vi "Servo and moisture.vi"() -> (0 "LOW MOISTURE":bool, 1 "INTERMEDIATE MOISTURE":bool, 2 "HIGH MOISTURE":bool, 3 "MOISTURE LEVEL(ppm)":dbl)   [LabVIEW 2013]
uses:
  <vilib>/myRIO/Common/Instrument Driver Framework/myRIO v1.0/PWM/vis/myRIO v1.1 Open PWM.vi
  <vilib>/myRIO/Common/Instrument Driver Framework/Utilities/vis/Validate Channels.vi
  <vilib>/myRIO/Common/Instrument Driver Framework/myRIO v1.0/PWM/vis/myRIO v1.0 Reserve PWM.vi
  <vilib>/myRIO/Common/Instrument Driver Framework/myRIO v1.0/PWM/vis/myRIO v1.0 Build MUX Configuration PWM.vi
  <vilib>/myRIO/Common/Instrument Driver Framework/myRIO v1.0/Resource Manager/vis/myRIO v1.0 Reserve Channel List.vi
  <vilib>/myRIO/Common/Instrument Driver Framework/myRIO v1.0/Resource Manager/vis/myRIO v1.0 Create Configuration List.vi
  <vilib>/myRIO/Common/Instrument Driver Framework/myRIO v1.0/Resource Manager/vis/myRIO v1.0 Reserve Channel.vi
  <vilib>/myRIO/Common/Instrument Driver Framework/myRIO v1.0/Resource Manager/vis/myRIO v1.0 Unreserve Channel.vi
  <vilib>/myRIO/Common/Instrument Driver Framework/myRIO v1.0/Resource Manager/vis/myRIO v1.0 Build Mutex Name.vi
  <vilib>/myRIO/Common/Instrument Driver Framework/myRIO v1.0/myRIO v1.1 Open.vi
  <vilib>/Utility/VariantDataType/GetNumericInfo.vi
  <vilib>/Utility/error.llb/Error Cluster From Error Code.vi
  <vilib>/myRIO/Common/Instrument Driver Framework/Utilities/vis/IO Manager.vi
  <vilib>/myRIO/Common/Instrument Driver Framework/Utilities/vis/Configuration Manager.vi
  <vilib>/myRIO/Common/Instrument Driver Framework/myRIO v1.0/Resource Manager/vis/myRIO v1.0 Configure IO.vi
  <vilib>/myRIO/Common/Instrument Driver Framework/myRIO v1.0/myRIO v1.0 Close.vi
  <vilib>/myRIO/Common/Instrument Driver Framework/myRIO v1.0/PWM/vis/myRIO v1.0 Write PWM.vi
  <vilib>/myRIO/Instrument Drivers/Onboard IO/PWM/PWM.lvlib
panel:
  in  "null offset":bool
  in  "freq [Hz] 2":dbl=50.0
  out "pulse width [ms] 2":dbl=1.5
  out "duty cycle [%] 2":dbl
  in  "null offset 2":bool
  out "offset [%FS] 2":dbl
  in  "PWM channel":tag="B/PWM0"
  in  "freq [Hz]":dbl=50.0
  out "pulse width [ms]":dbl=1.5
  out "duty cycle [%]":dbl
  out "offset [%FS]":dbl
  out "x+y":dbl
  # "SERVO"
  # "MOISTURE"
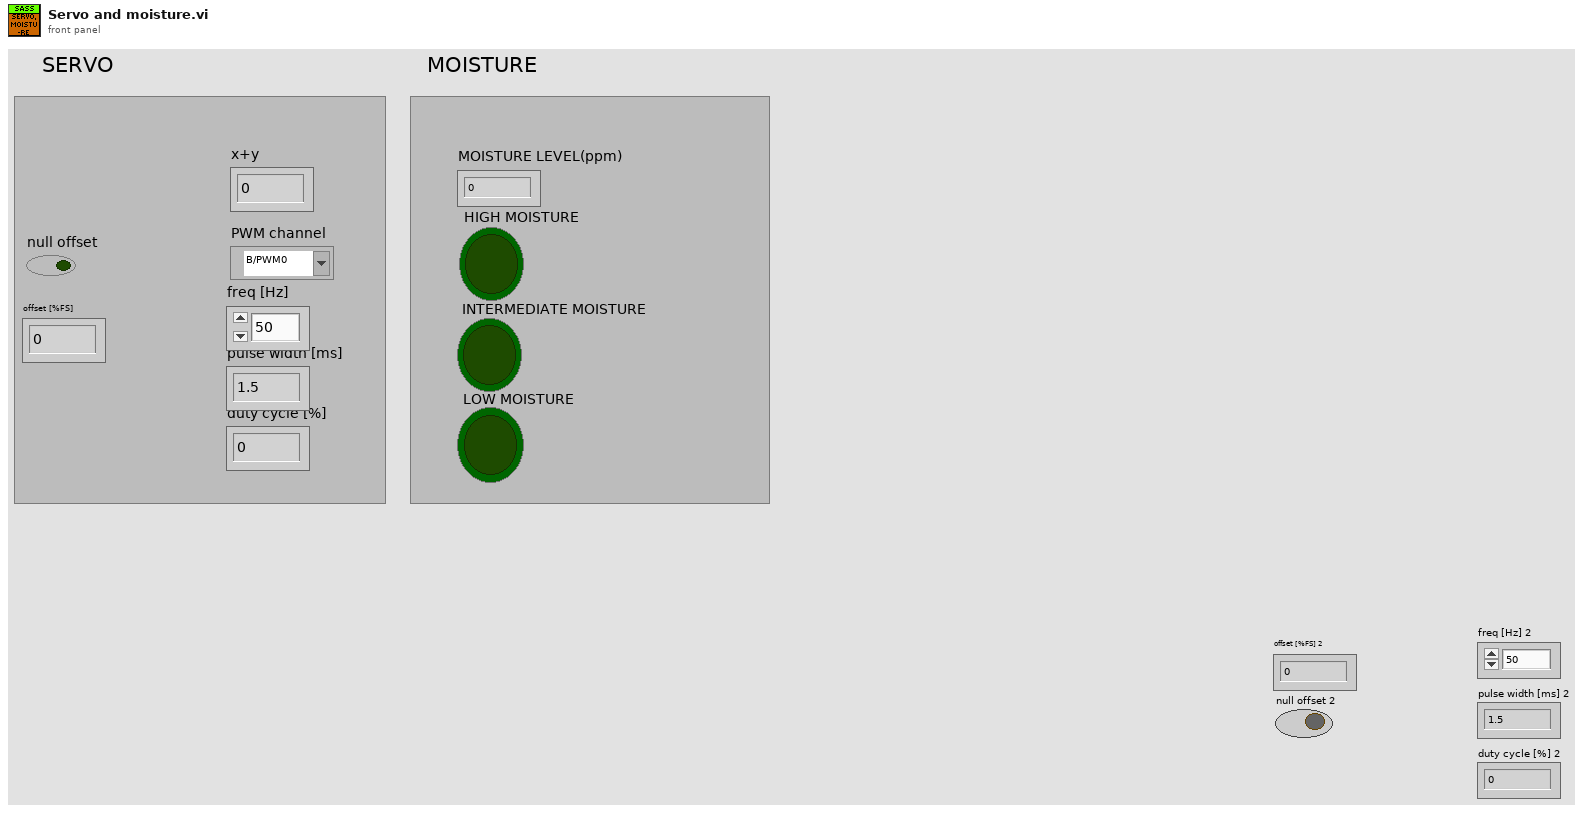
[diagram p1: front panel]
types:
  T1 = typedef "PWM.lvlib/PWM Reference.ctl" = cluster{"myRIO Reference":T2, "PWM Channels Enum":T6, "PWM Configuration":T7}
  T2 = typedef "myRIO Generic Hardware Reference.ctl" = cluster{"myRIO Model":T3, "myRIO Hardware Reference":T4}
  T3 = typedef "Hardware Version Enum.ctl" = enum16{"Unknown", "myRIO-1900", "myRIO-1950"}
  T4 = typedef "myRIO v1.0 Reference.ctl" = cluster{"Generic FPGA Reference":T5, "Allow multiple opens":bool}
  T5 = typedef "Generic FPGA Reference.ctl" = refnum<k20>
  T6 = typedef "PWM Channels Enum.ctl" = enum16{"Not Connected", "C/PWM0", "C/PWM1", "A/PWM0", "A/PWM1", "A/PWM2", "B/PWM0", "B/PWM1", "B/PWM2"}
  T7 = typedef "PWM.lvlib/PWM Configuration.ctl" = cluster{"Frequency":dbl, "Duty Cycle":dbl}
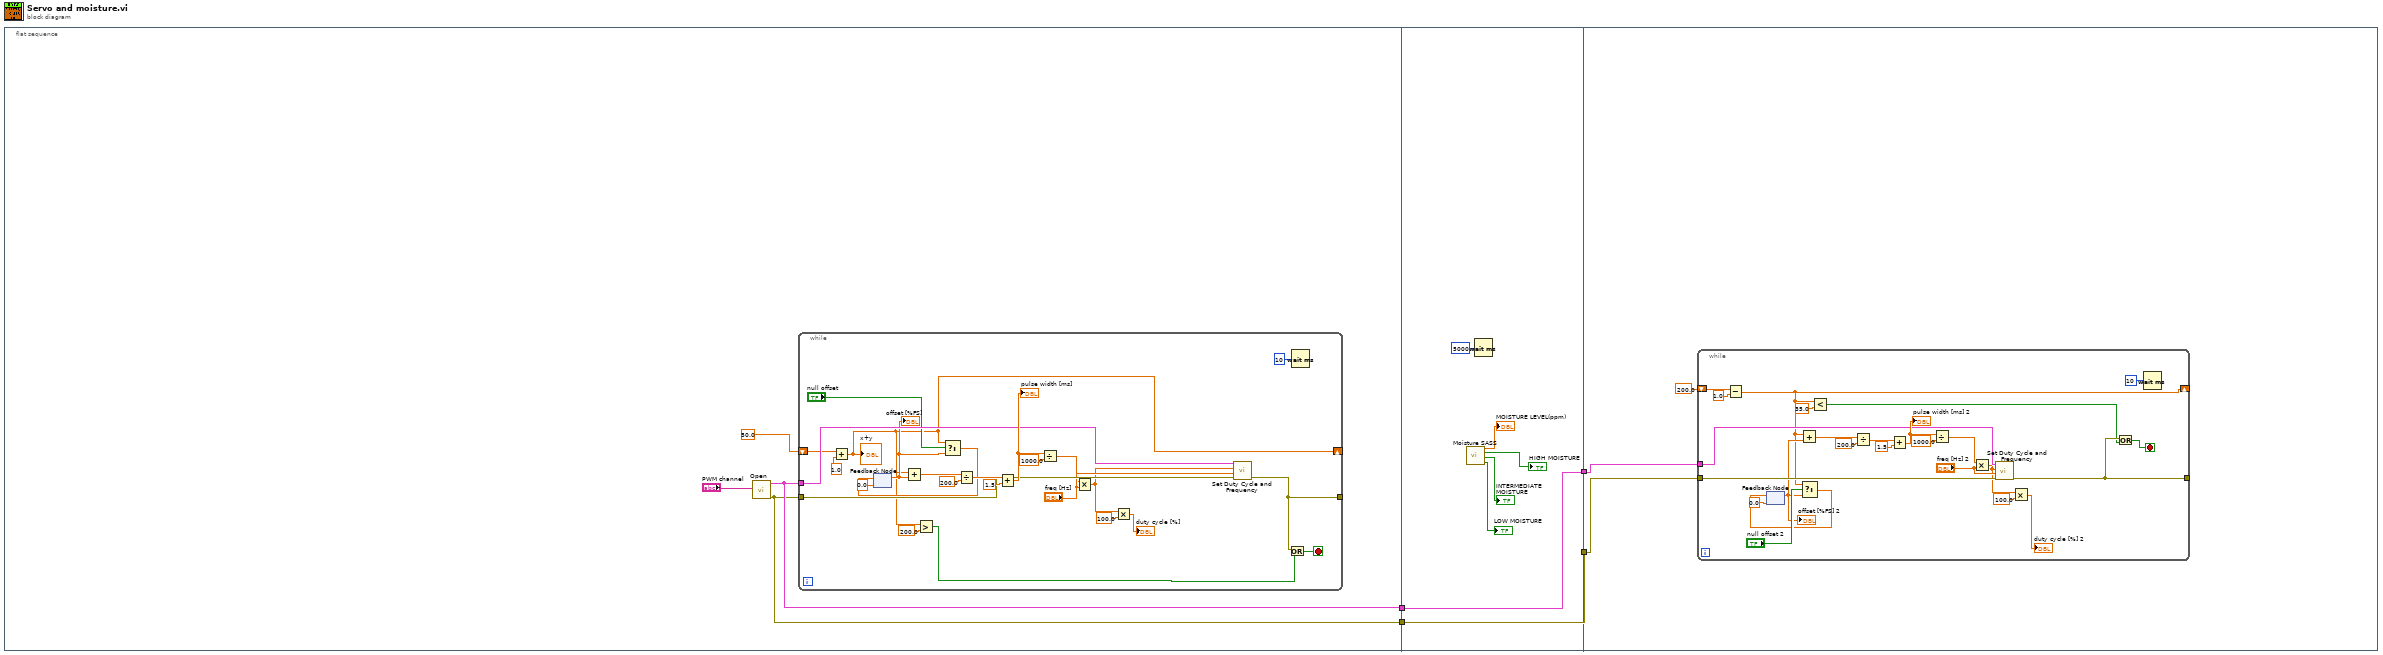
[diagram p0: block diagram]
diagram:
  n1 = flat-sequence {
    tunnel: [w6] -> w3
    tunnel: [w5] -> w1
    tunnel: [w34] -> w4
    tunnel: w3 -> [w34]
    tunnel: [w39] -> w2
    tunnel: w1 -> [w39]
    tunnel: w4 -> [w42]
    tunnel: w2 -> [w41]
    frame #0 {
      n2 = call <vilib>:"Open.vi"("Channel Name"="PWM channel") -> ("error out"=w5:errorcluster, "PWM Ref Out"=w6:T1)  [unwired: 9 in]
      n3 = while {
        tunnel: w6 -> [w26]
        tunnel: w5 -> [w25]
        tunnel: [w23] -> _
        shift-right: [w11] -> _
        shift-left: 50.0 ("Numeric Control") -> [w12]
        stop <- w33 stop-if-true
        n4 = Add(x=w12, y=1.0) -> (x+y=w11:dbl)
        "x+y" <- w11
        n5 = feedback #1(0.0 ("position [%FS]")) -> (w19:dbl)
        "offset [%FS]" <- w19
        n6 = Add(x=w11, y=w19) -> (x+y=w20:dbl)
        n7 = Greater?(x=w11, y=200.0) -> (0:w9:bool)
        n8 = Select(t=w11, s="null offset", f=w19) -> (s? t:f=w21:dbl)
        n9 = feedback-in #1(w21) -> ()
        n10 = Divide(x=w20, y=200.0) -> (x/y=w30:dbl)
        n11 = Add(x=w30, y=1.5) -> (x+y=w28:dbl)
        "pulse width [ms]" <- w28
        n12 = Divide(x=w28, y=1000.0) -> (x/y=w18:dbl)
        n13 = Multiply(x=w18, y="freq [Hz]") -> (x*y=w15:dbl)
        n14 = Multiply(x=w15, y=100.0) -> (x*y=→"duty cycle [%]":dbl)
        n15 = call <vilib>:"Set Duty Cycle and Frequency.vi"("error in (no error)"=w25, "Frequency (Hz)"="freq [Hz]", "Duty Cycle (0-1)"=w15, "PWM Ref In"=w26) -> ("error out"=w23:errorcluster)  [unwired: 5 in, 1 out]
        n16 = Or(x=w23, y=w9) -> (x .or. y?=w33:bool)
        n17 = Wait (ms)(milliseconds to wait=u32 10) -> ()  [unwired: 1 out]
      }
    }
    frame #1 {
      n18 = call "Moisture SASS.vi"() -> ("LOW MOISTURE"=→"LOW MOISTURE":bool, "INTERMEDIATE MOISTURE"=→"INTERMEDIATE MOISTURE":bool, "HIGH MOISTURE"=→"HIGH MOISTURE":bool, "MOISTURE LEVEL(ppm)"=→"MOISTURE LEVEL(ppm)":dbl)  [unwired: 8 in]
      n19 = Wait (ms)(milliseconds to wait=u32 5000) -> ()  [unwired: 1 out]
    }
    frame #2 {
      n20 = while {
        tunnel: w42 -> [w61]
        tunnel: w41 -> [w60]
        tunnel: [w58] -> _
        shift-right: [w46] -> _
        shift-left: 200.0 -> [w47]
        stop <- w68 stop-if-true
        n21 = Subtract(x=w47, y=1.0) -> (x-y=w46:dbl)
        n22 = feedback #2(0.0 ("position [%FS]")) -> (w54:dbl)
        "offset [%FS] 2" <- w54
        n23 = Add(x=w46, y=w54) -> (x+y=w55:dbl)
        n24 = Select(t=w46, s="null offset 2", f=w54) -> (s? t:f=w56:dbl)
        n25 = feedback-in #2(w56) -> ()
        n26 = Less?(x=w46, y=35.0) -> (x < y?=w44:bool)
        n27 = Divide(x=w55, y=200.0) -> (x/y=w65:dbl)
        n28 = Add(x=w65, y=1.5) -> (x+y=w63:dbl)
        "pulse width [ms] 2" <- w63
        n29 = Divide(x=w63, y=1000.0) -> (x/y=w53:dbl)
        n30 = Multiply(x=w53, y="freq [Hz] 2") -> (x*y=w50:dbl)
        n31 = call <vilib>:"Set Duty Cycle and Frequency.vi"("error in (no error)"=w60, "Frequency (Hz)"="freq [Hz] 2", "Duty Cycle (0-1)"=w50, "PWM Ref In"=w61) -> ("error out"=w58:errorcluster)  [unwired: 5 in, 1 out]
        n32 = Multiply(x=w50, y=100.0) -> (x*y=→"duty cycle [%] 2":dbl)
        n33 = Or(x=w58, y=w44) -> (x .or. y?=w68:bool)
        n34 = Wait (ms)(milliseconds to wait=u32 10) -> ()  [unwired: 1 out]
      }
    }
  }
